vi "Testeo de adquisición de imagenes.vi"() -> ()   [LabVIEW 2021]
uses:
  <vilib>/vision/Pattern Matching.llb/IMAQ GM Match Report.ctl
panel:
  out "Matches (Pattern Matching 1)":T1[](array[typedef]) {"Correlation Score" format="%.2f"; "Target Template Curve Score" format="%.2f"; "Template Target Curve Score" format="%.2f"; "Bounding Box"."y" format="%.2f"; "Bounding Box"."x" format="%.2f"; "Position"."y" format="%.2f"; "Position"."x" format="%.2f"; "Score" format="%.2f"; "Scale" format="%.2f"; "Angle" format="%.2f"; "Occlusion %" format="%.2f"}
  out "Image Out":T2(plugin-control)
  in  "stop":bool
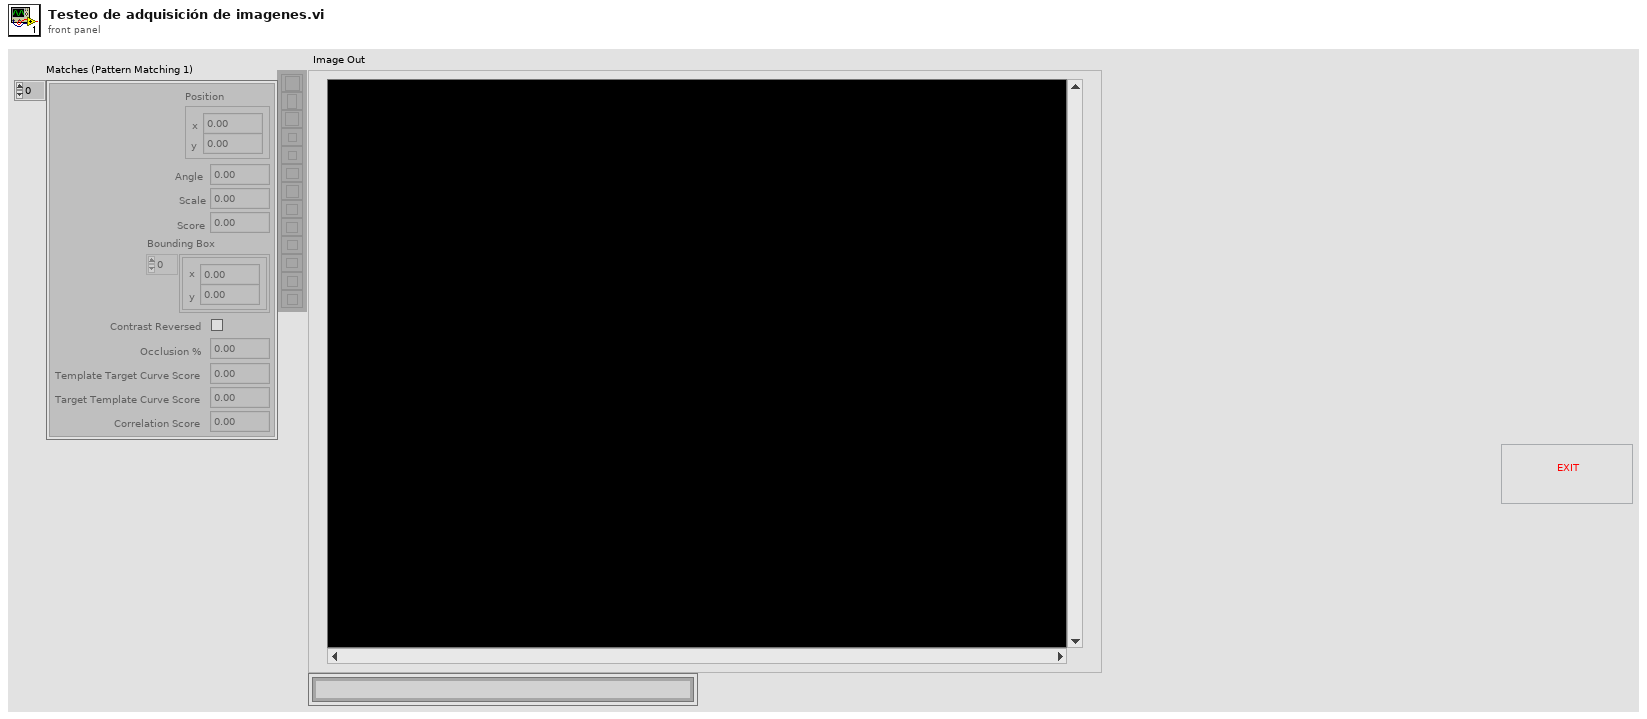
[diagram p1: front panel]
types:
  T1 = typedef "IMAQ GM Match Report.ctl" = cluster{"Position":cluster{"x":sgl, "y":sgl}, "Angle":sgl, "Scale":sgl, "Score":sgl, "Bounding Box":cluster{"x":sgl, "y":sgl}[], "Contrast Reversed":bool, "Occlusion %":sgl, "Template Target Curve Score":sgl, "Target Template Curve Score":sgl, "Correlation Score":sgl}
  T2 = typedef "IMAQ Image.ctl" = refnum<image>
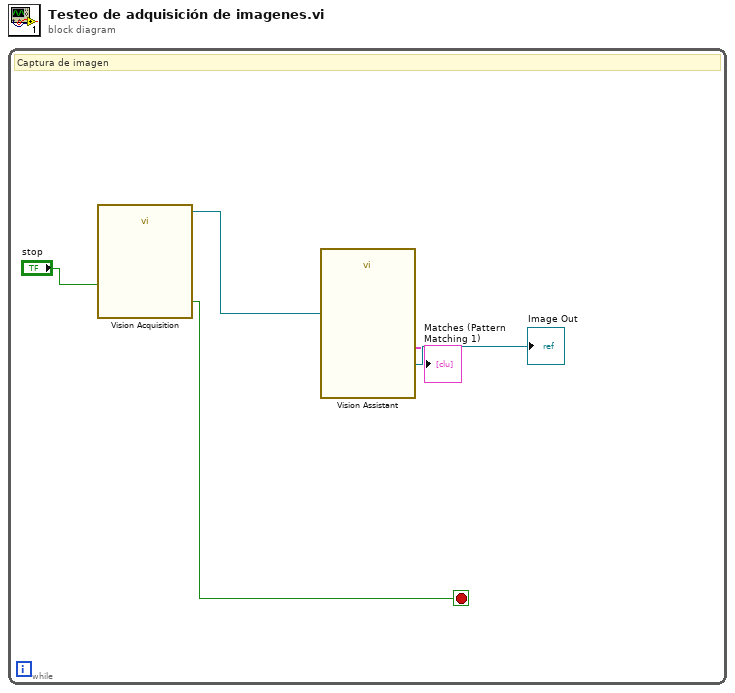
[diagram p0: block diagram]
diagram:
  n1 = while {
    stop <- w5 stop-if-true
    # "Captura de imagen"
    n2 = call "Vision Acquisition"("Stop (F)"="stop") -> ("Image Out"=w3:T2, "Stopped"=w5:bool)  [unwired: 24 in, 1 out]
    n3 = call "Vision Assistant"("Image In"=w3) -> ("Image Out"=→"Image Out":T2, "Matches (Pattern Matching 1)"=→"Matches (Pattern Matching 1)":T1[])  [unwired: 23 in, 2 out]
  }
